vi "TrimXY.vi"(5 "X-max":dbl, 7 "X-min":dbl, 8 "Y-max":dbl, 9 "Y-min":dbl, 10 "Array In":dbl[][](array[numeric]), 11 "Trim data":bool caption="Scan") -> (2 "Array Trim Out":dbl[][](array[numeric]))   [LabVIEW 2018]
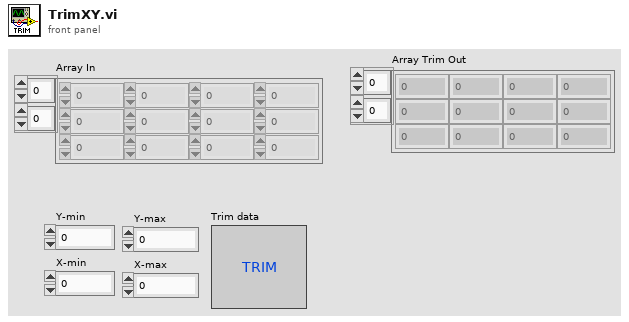
[diagram p1: front panel]
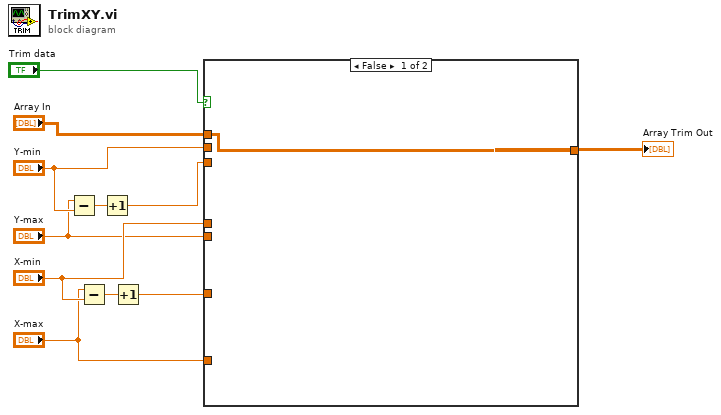
[diagram p0: block diagram]
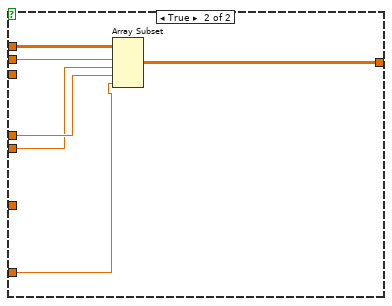
[diagram p2: hidden frame]
diagram:
  n1 = Subtract(x="Y-max", y="Y-min") -> (x-y=w7:dbl)
  n2 = Subtract(x="X-max", y="X-min") -> (x-y=w5:dbl)
  n3 = Increment(x=w7) -> (x+1=w6:dbl)
  n4 = Increment(x=w5) -> (x+1=w4:dbl)
  n5 = case shown="False" "Trim data" {
    tunnel: "Array In" -> [w12 w15]
    tunnel: [w12 w16] -> w10
    tunnel: "Y-min" -> [_ w18]
    tunnel: w6 -> [_ _]
    tunnel: "X-min" -> [_ w17]
    tunnel: w4 -> [_ _]
    tunnel: "Y-max" -> [_ w14]
    tunnel: "X-max" -> [_ w13]
    frame False {
    }
    frame True {
      n6 = Array Subset(array=w15, index (row)=w18, length (row)=w14, index (col)=w17, length (col)=w13) -> (w16:dbl[][])
    }
  }
  "Array Trim Out" <- w10
